vi "Find keeper counts.vi"(10 "Support Map":map{i32, set{i32}}(c390), 11 "Brick Map":map{i32, T2[]}(c390)) -> (3 "Keep Map":map{i32, T1}(c390))   [LabVIEW 2023]
uses:
  Cluster_Node.ctl
  Cluster_Dependencies.ctl
  <vilib>/Utility/miscctls.llb/LVMapReplaceAction.ctl
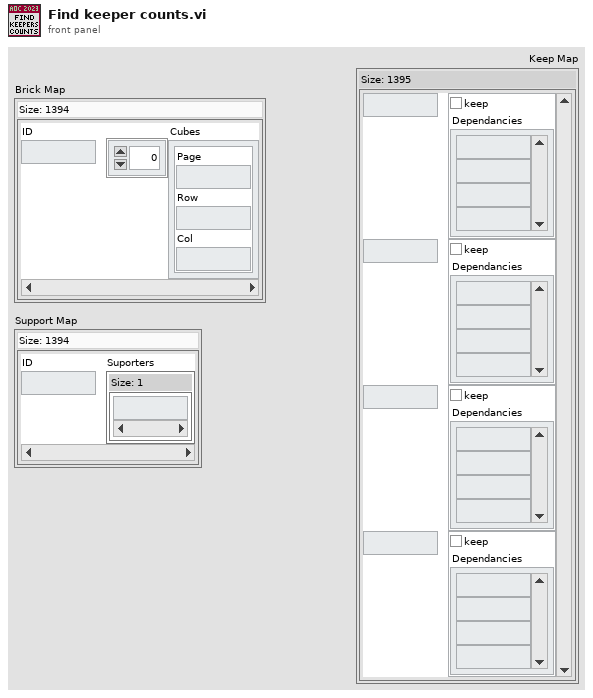
[diagram p1: front panel]
types:
  T1 = typedef "Cluster_Dependencies.ctl" = cluster{"keep":bool, "Dependancies":i32[]}
  T2 = typedef "Cluster_Node.ctl" = cluster{"Page":i32, "Row":i32, "Col":i32}
  T3 = typedef "LVMapReplaceAction.ctl" = enum32{"Modify Entry only if found", "Add or Modify Entry", "Delete Entry"}
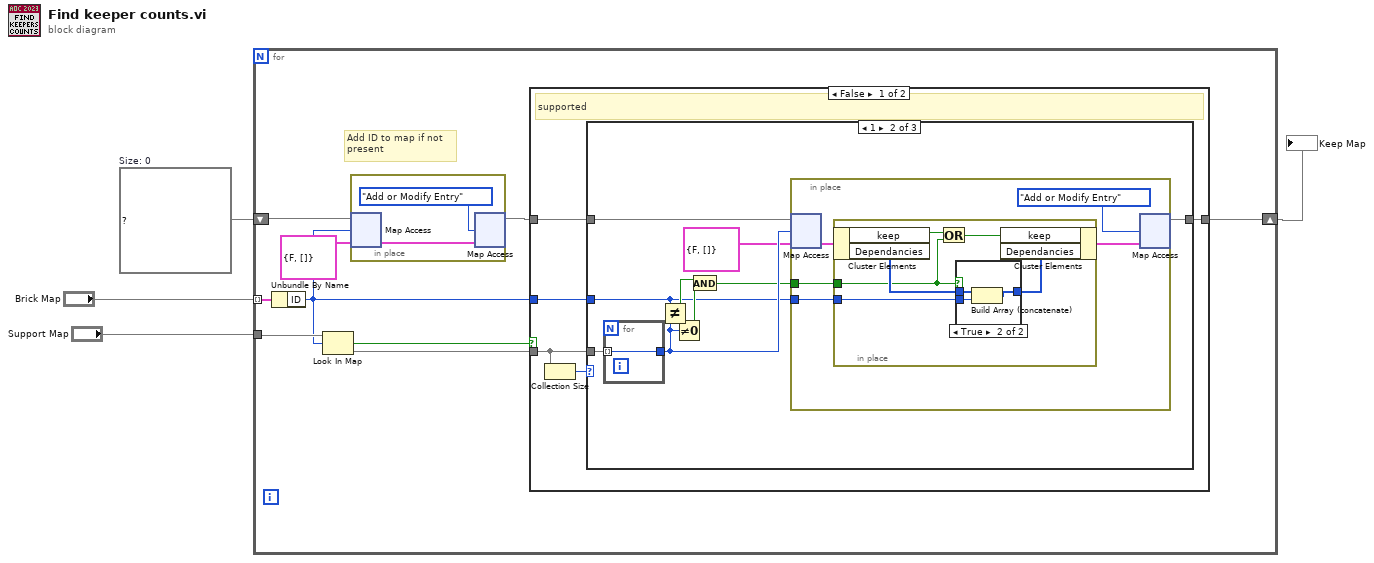
[diagram p0: block diagram]
diagram:
  w2 = map{i32, T1} {}  # Size: 0
  n1 = for {
    tunnel: "Brick Map" -> [w13] mode=indexing
    tunnel: "Support Map" -> [w12]
    shift-right: [w11] -> w1
    shift-left: w2 -> [w10]
    # "Add ID to map if not\npresent"
    n2 = Unbundle By Name(w13) -> ("ID"=w9:i32)
    n3 = Look In Map(map=w12, key=w9) -> (key not found?=w8:bool, value=w7:set{i32})  [unwired: 1 in]
    n4 = in-place {
      n5 = in-place-map #1(w10, w9, T1 {"keep"=FALSE, "Dependancies"=[]} ("Dependancies")) -> (w14:T1)  [unwired: 1 out]
      n6 = in-place-map #1(w14, LVMapReplaceAction."Add or Modify Entry" ("action")) -> (w6:map{i32, T1})  [unwired: 2 out]
    }
    n7 = case shown="False" w8 {
      tunnel: w7 -> [w19 _]
      tunnel: w6 -> [w18 w48]
      tunnel: w9 -> [w17 _]
      tunnel: [w16 w48] -> w11
      frame False {
        # "supported"
        n8 = Collection Size(1:w19) -> (0:w20:i32)
        n9 = case shown="1" w20 {
          tunnel: w19 -> [_ w30 _]
          tunnel: w18 -> [w21 w29 w47]
          tunnel: w17 -> [_ w22 _]
          tunnel: [w21 w28 w47] -> w16
          frame ..0 {
            # "Never supoosed to happen"
            # "every ID should have support"
          }
          frame 1 {
            n10 = for {
              tunnel: w30 -> [w46] mode=indexing
              tunnel: [w46] -> w27
            }
            n11 = Not Equal?(x=w22, y=w27) -> (x != y?=w26:bool)
            n12 = Not Equal To 0?(x=w27) -> (x != 0?=w25:bool)
            n13 = And(x=w26, y=w25) -> (x .and. y?=w24:bool)
            n14 = in-place {
              in-place-border: w24 -> [w34]
              in-place-border: w22 -> [w31]
              n15 = in-place-map #2(w29, w27, T1 {"keep"=FALSE, "Dependancies"=[]} ("Dependancies")) -> (w33:T1)  [unwired: 1 out]
              n16 = in-place {
                in-place-border: w34 -> [w37]
                in-place-border: w31 -> [w36]
                n17 = in-place-cluster #3(w33) -> ("keep"=w41:bool, "Dependancies"=w39:i32[])
                n18 = Or(x=w41, y=w37) -> (x .or. y?=w40:bool)
                n19 = case shown="True" w37 {
                  tunnel: w39 -> [w42 w45]
                  tunnel: [w42 w44] -> w38
                  tunnel: w36 -> [_ w43]
                  frame False {
                  }
                  frame True {
                    n20 = Build Array (concatenate)(w45, w43) -> (w44:i32[])
                  }
                }
                n21 = in-place-cluster #3("keep"=w40, "Dependancies"=w38) -> (w32:T1)
              }
              n22 = in-place-map #2(w32, LVMapReplaceAction."Add or Modify Entry" ("action")) -> (w28:map{i32, T1})  [unwired: 2 out]
            }
          }
          frame 2.. {
            # "Has multiple supporters"
          }
        }
      }
      frame True {
        # "All should be supported \nso this should never happen"
        # "not supported"
      }
    }
  }
  "Keep Map" <- w1
